vi "FPGA_Master.vi"() -> ()   [LabVIEW 2019]
panel:
  out "Error ?":bool=TRUE
  out "Start sequence?":bool=TRUE
  out "NE cluster":T1
  out "Input Signal / mV":fxp<+/-,19,14> format="%.3g"
  out "Filtered Input":i16(graph)
  out "Filtered Input 2":fxp<+/-,16,16>
  in  "override noise eater?":bool
  in  "Setpoint (H)":fxp<+/-,16,16>
  out "Control Signal / mV":fxp<+/-,19,14> format="%.3g"
  out "Control Signal":i16(graph)
  in  "Setpoint (L)":fxp<+/-,16,16> format="%.3f"
  in  "High power":bool
  in  "Controller output range":T2={"Output high"=10.0, "Output low"=-10.0}
  in  "PID gains":T3={"Proportional gain Kc"=0.0, "Integral time Ti [min]"=2.0, "Derivative time Td [min]"=0.0}
  in  "Reinitialise controller":bool
  out "DIO cluster":T4
  out "AO cluster":T5
  in  "AO7":i16
  in  "AO6":i16
  in  "AO5":i16
  in  "AO4 on":i16
  in  "AO4 off":i16
  in  "AO1 off":i16
  in  "AO1 on":i16
  in  "AO2 off":i16
  in  "AO2 on":i16
  in  "AO3 off":i16
  in  "AO3 on":i16
  in  "AO4":bool
  in  "AO1":bool
  in  "AO3":bool
  in  "AO2":bool
  in  "D31":bool
  in  "D30":bool
  in  "D29":bool
  in  "D28":bool
  in  "D27":bool
  in  "D26":bool
  in  "D25":bool
  in  "D24":bool
  in  "D23":bool
  in  "D22":bool
  in  "D21":bool
  in  "D20":bool
  in  "D19":bool
  in  "D18":bool
  in  "D17":bool
  in  "D16":bool
  in  "D15":bool
  in  "D14":bool
  in  "D13":bool
  in  "D12":bool
  in  "DIO11":bool
  in  "DIO5":bool
  in  "DIO4":bool
  in  "dds/ag":bool
  in  "DIO8":bool
  in  "DIO9":bool
  in  "DIO7":bool
  in  "DIO6":bool
  in  "EOM":bool
  in  "Microwave":bool
  in  "DIO10":bool
  in  "AOM":bool
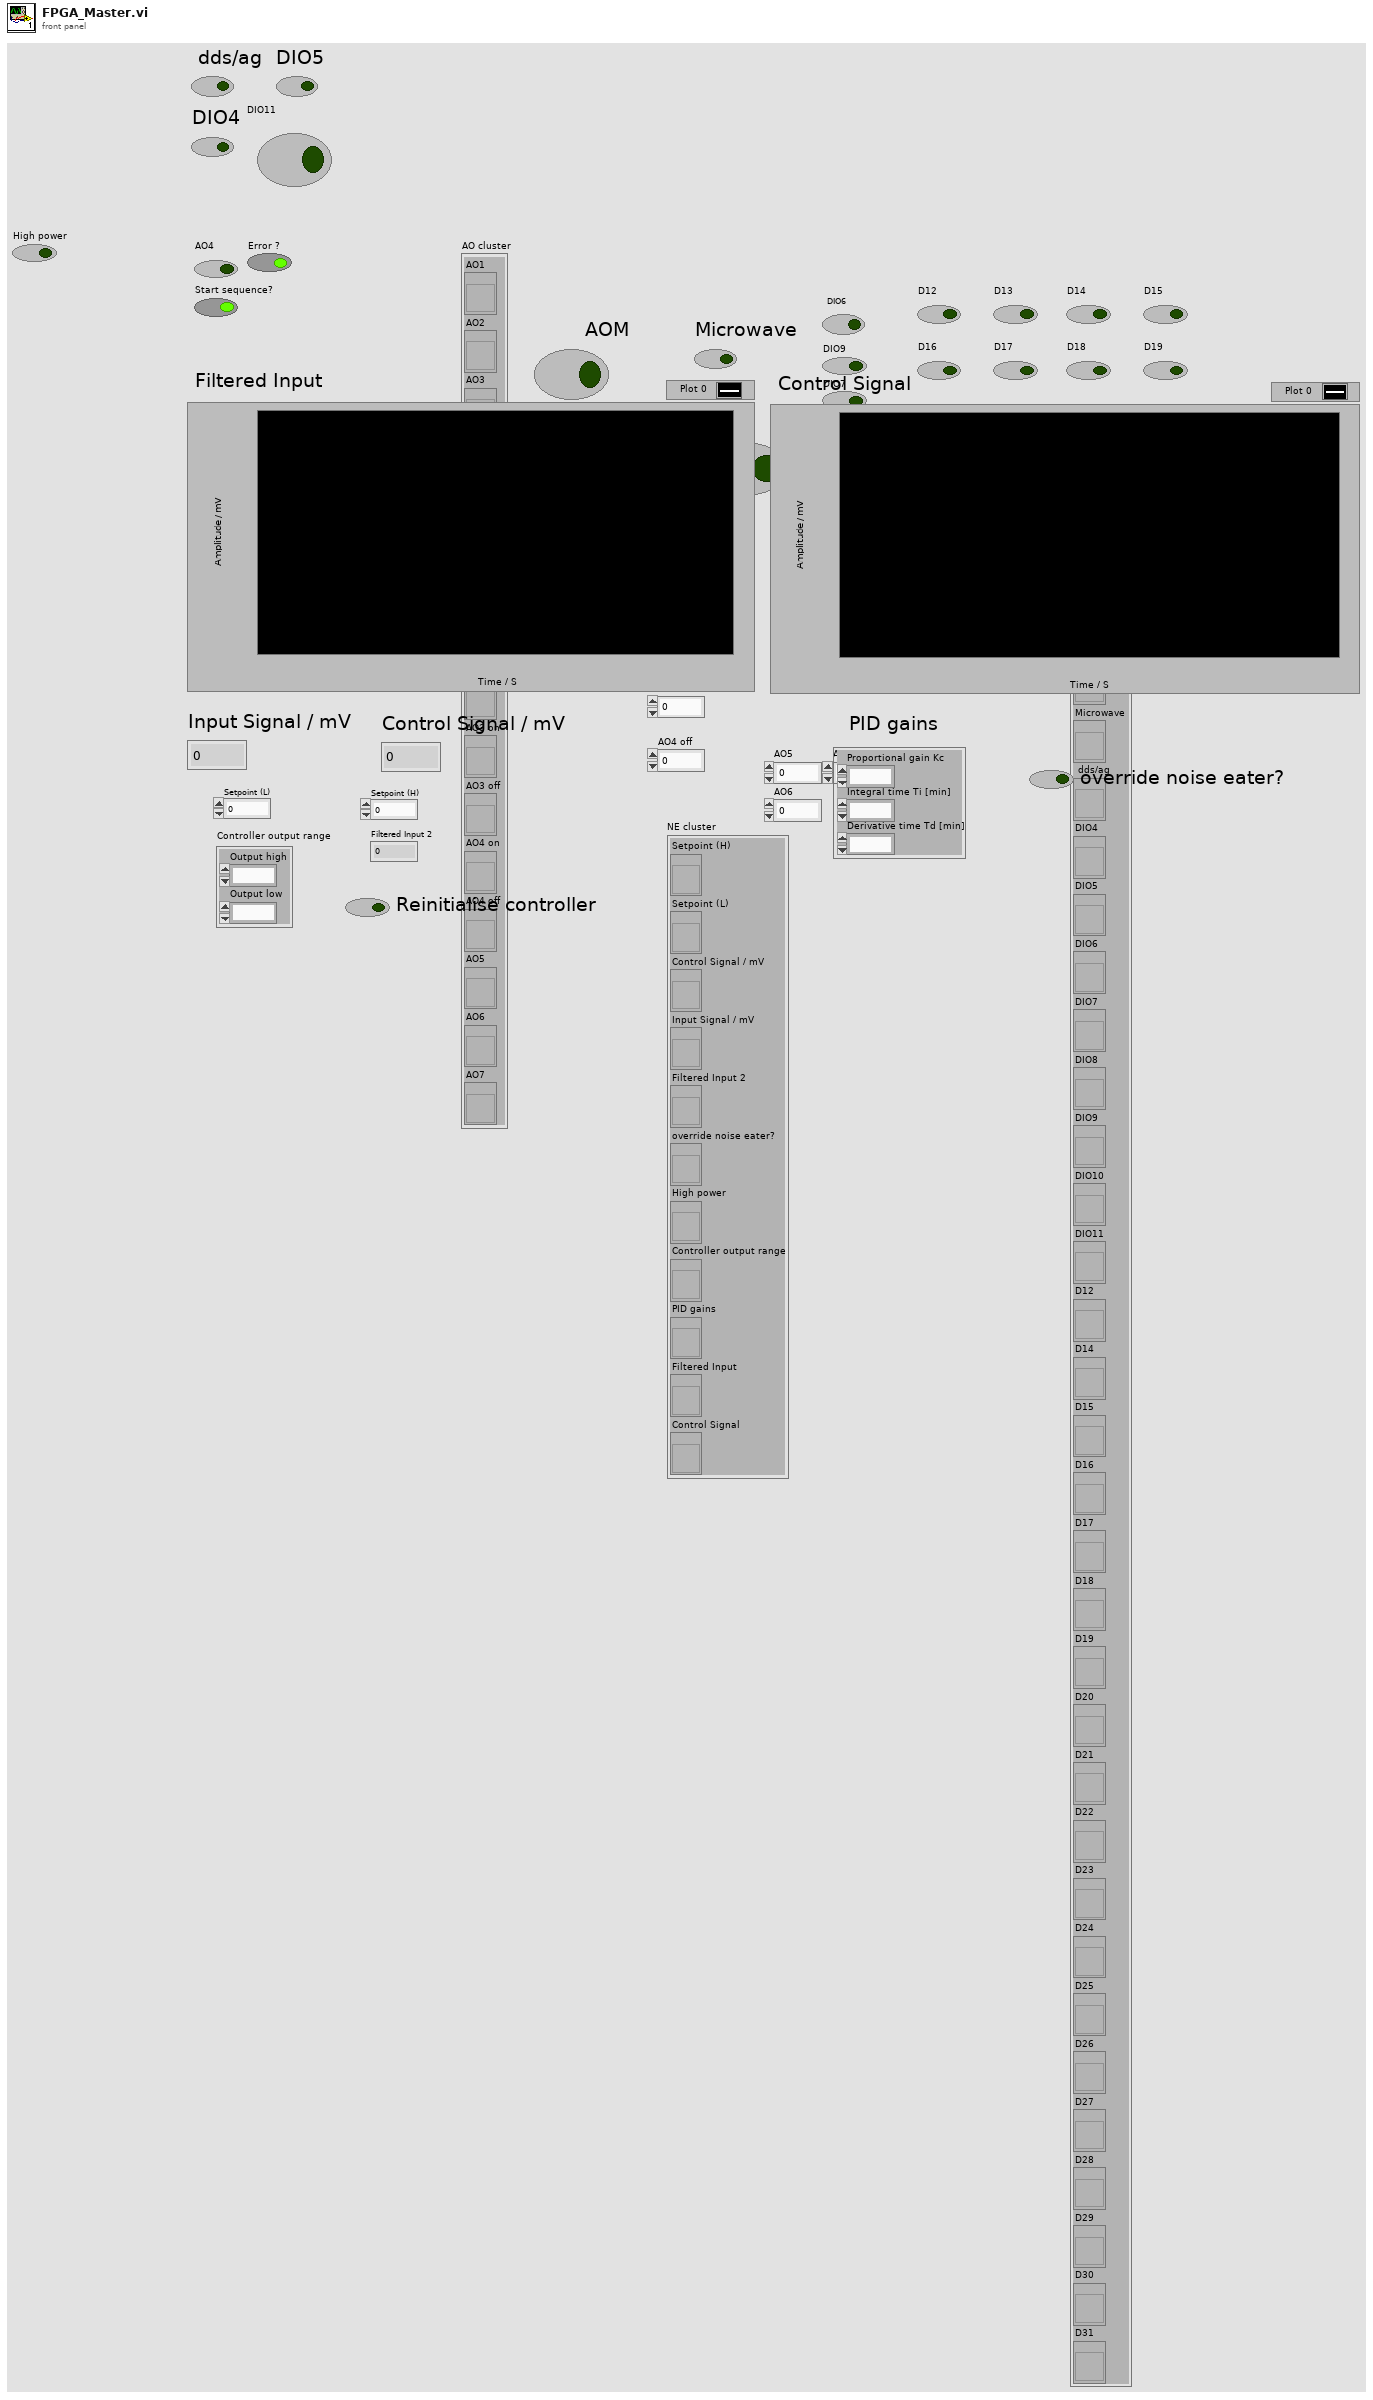
[diagram p1: front panel]
types:
  T1 = cluster{"Setpoint (H)":refnum<vi>, "Setpoint (L)":refnum<vi>, "Control Signal / mV":refnum<vi>, "Input Signal / mV":refnum<vi>, "Filtered Input 2":refnum<vi>, "override noise eater?":refnum<vi>, "High power":refnum<vi>, "Controller output range":refnum<vi>, "PID gains":refnum<vi>, "Filtered Input":refnum<vi>, "Control Signal":refnum<vi>}
  T2 = cluster{"Output high":fxp<+/-,16,16>, "Output low":fxp<+/-,16,16>}
  T3 = cluster{"Proportional gain Kc":fxp<+/-,16,8>, "Integral time Ti [min]":fxp<+/-,16,8>, "Derivative time Td [min]":fxp<+/-,16,8>}
  T4 = cluster{"AOM":refnum<vi>, "EOM":refnum<vi>, "Microwave":refnum<vi>, " dds/ag":refnum<vi>, "DIO4":refnum<vi>, "DIO5":refnum<vi>, "DIO6":refnum<vi>, "DIO7":refnum<vi>, "DIO8":refnum<vi>, "DIO9":refnum<vi>, "DIO10":refnum<vi>, "DIO11":refnum<vi>, "D12":refnum<vi>, "D14":refnum<vi>, "D15":refnum<vi>, "D16":refnum<vi>, "D17":refnum<vi>, "D18":refnum<vi>, "D19":refnum<vi>, "D20":refnum<vi>, "D21":refnum<vi>, "D22":refnum<vi>, "D23":refnum<vi>, "D24":refnum<vi>, "D25":refnum<vi>, "D26":refnum<vi>, "D27":refnum<vi>, "D28":refnum<vi>, "D29":refnum<vi>, "D30":refnum<vi>, "D31":refnum<vi>}
  T5 = cluster{"AO1":refnum<vi>, "AO2":refnum<vi>, "AO3":refnum<vi>, "AO4":refnum<vi>, "AO1 on":refnum<vi>, "AO1 off":refnum<vi>, "AO2 on":refnum<vi>, "AO2 off":refnum<vi>, "AO3 on":refnum<vi>, "AO3 off":refnum<vi>, "AO4 on":refnum<vi>, "AO4 off":refnum<vi>, "AO5":refnum<vi>, "AO6":refnum<vi>, "AO7":refnum<vi>}
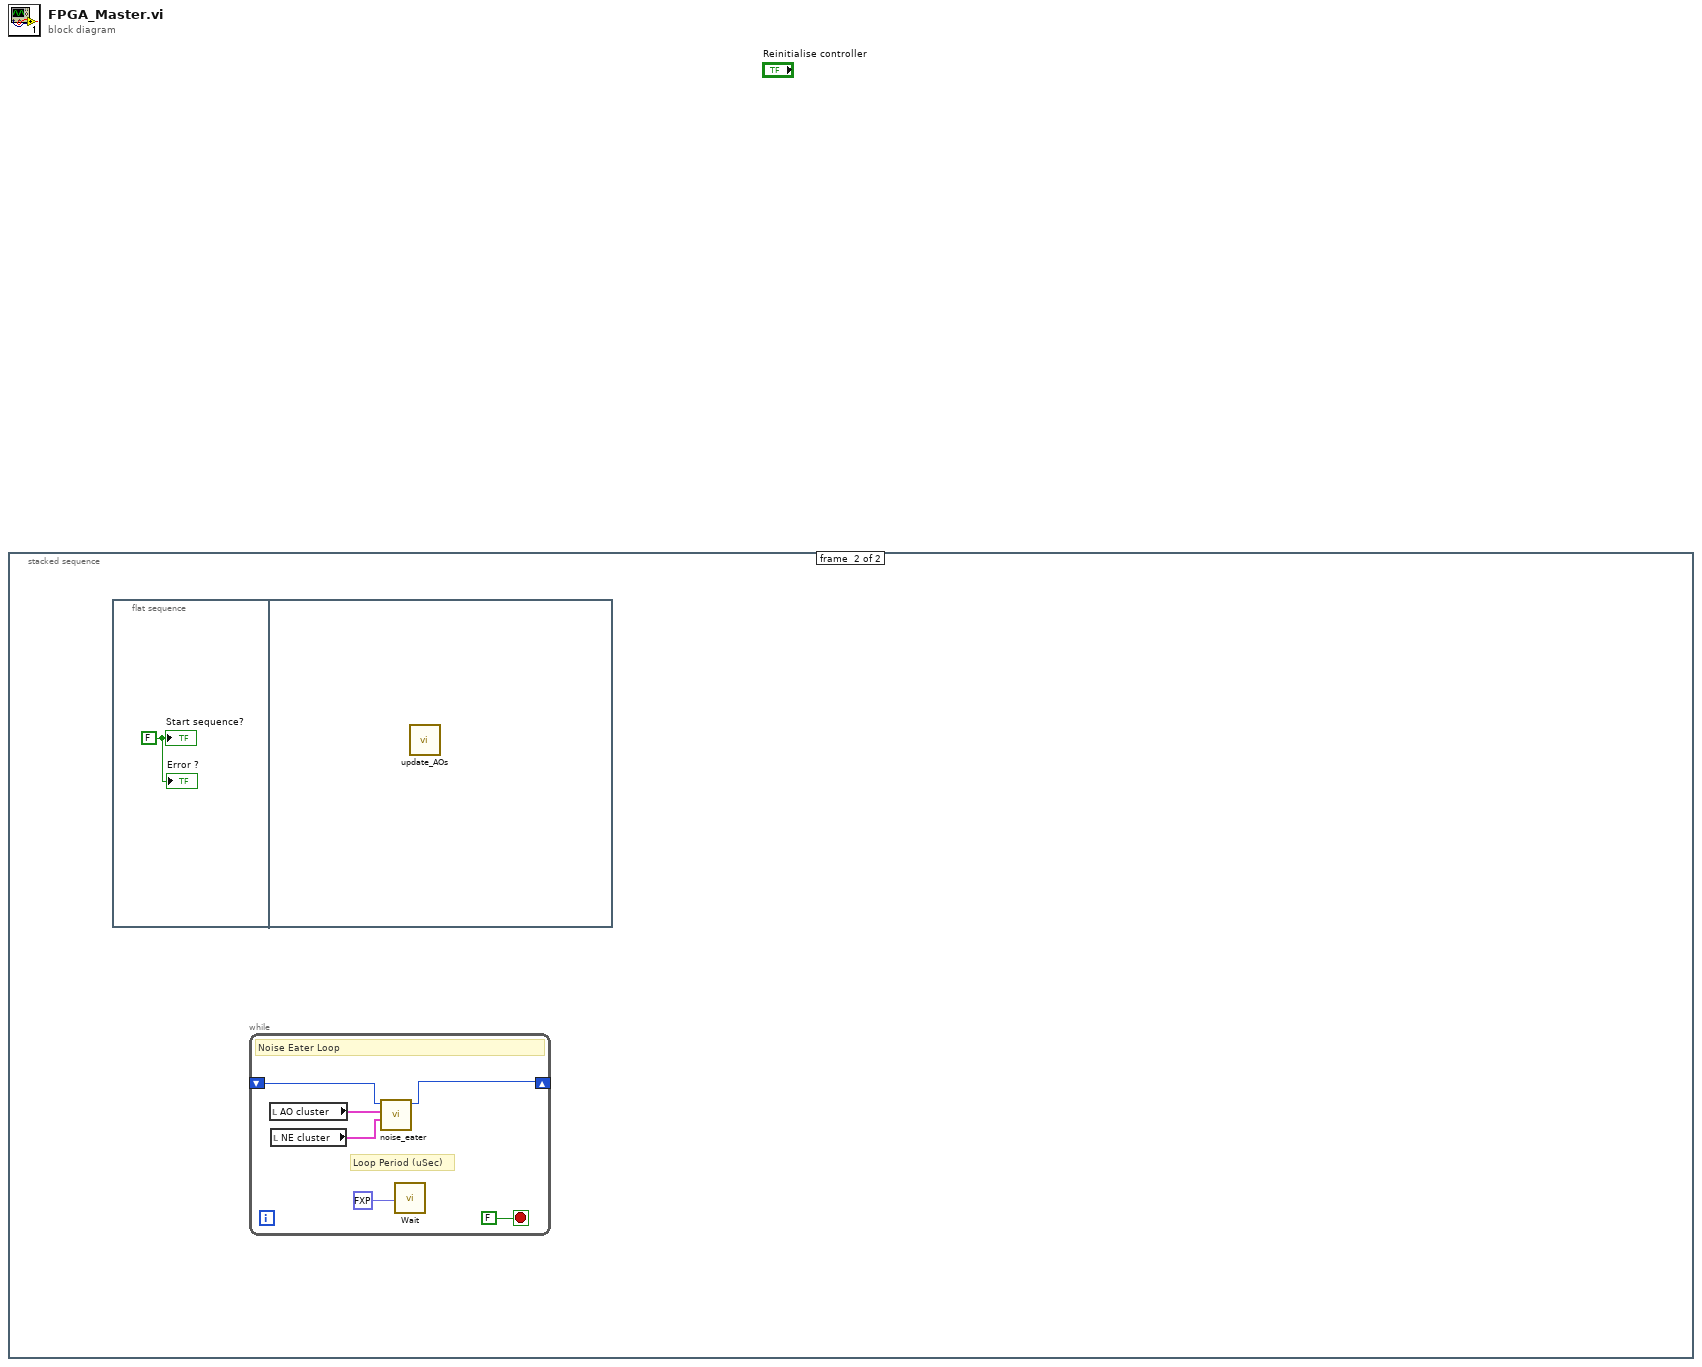
[diagram p0: block diagram]
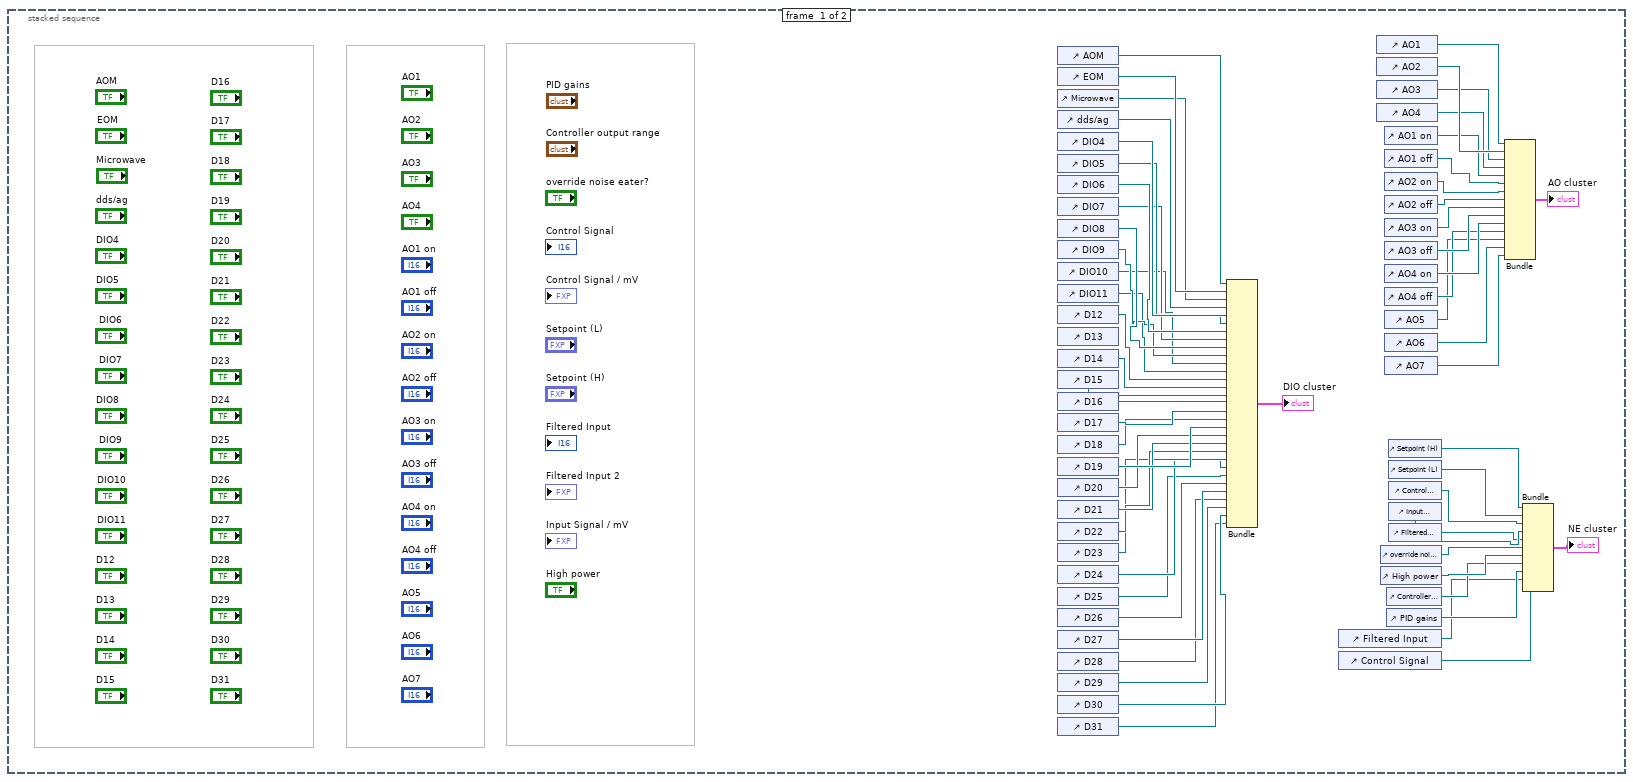
[diagram p2: hidden frame]
diagram:
  n1 = stacked-sequence {
    frame #0 {
      n2 = control-ref of="AOM"() -> (w44:refnum<vi>)
      n3 = control-ref of="EOM"() -> (w43:refnum<vi>)
      n4 = control-ref of="Microwave"() -> (w42:refnum<vi>)
      n5 = control-ref of="dds/ag"() -> (w41:refnum<vi>)
      n6 = control-ref of="DIO4"() -> (w40:refnum<vi>)
      n7 = control-ref of="DIO5"() -> (w39:refnum<vi>)
      n8 = control-ref of="DIO6"() -> (w38:refnum<vi>)
      n9 = control-ref of="DIO7"() -> (w37:refnum<vi>)
      n10 = control-ref of="DIO8"() -> (w36:refnum<vi>)
      n11 = control-ref of="DIO9"() -> (w35:refnum<vi>)
      n12 = control-ref of="DIO10"() -> (w34:refnum<vi>)
      n13 = control-ref of="DIO11"() -> (w33:refnum<vi>)
      n14 = control-ref of="D12"() -> (w32:refnum<vi>)
      n15 = control-ref of="D13"() -> ()  [unwired: 1 out]
      n16 = control-ref of="D14"() -> (w31:refnum<vi>)
      n17 = control-ref of="D15"() -> (w30:refnum<vi>)
      n18 = control-ref of="D16"() -> (w29:refnum<vi>)
      n19 = control-ref of="D17"() -> (w28:refnum<vi>)
      n20 = control-ref of="D18"() -> (w27:refnum<vi>)
      n21 = control-ref of="D19"() -> (w26:refnum<vi>)
      n22 = control-ref of="D20"() -> (w25:refnum<vi>)
      n23 = control-ref of="D21"() -> (w24:refnum<vi>)
      n24 = control-ref of="D22"() -> (w23:refnum<vi>)
      n25 = control-ref of="D23"() -> (w22:refnum<vi>)
      n26 = control-ref of="D24"() -> (w21:refnum<vi>)
      n27 = control-ref of="D25"() -> (w20:refnum<vi>)
      n28 = control-ref of="D26"() -> (w19:refnum<vi>)
      n29 = control-ref of="D27"() -> (w18:refnum<vi>)
      n30 = control-ref of="D28"() -> (w17:refnum<vi>)
      n31 = control-ref of="D29"() -> (w16:refnum<vi>)
      n32 = control-ref of="D30"() -> (w15:refnum<vi>)
      n33 = control-ref of="D31"() -> (w14:refnum<vi>)
      n34 = Bundle("AOM"=w44, "EOM"=w43, "Microwave"=w42, "dds/ag"=w41, "DIO4"=w40, "DIO5"=w39, "DIO6"=w38, "DIO7"=w37, "DIO8"=w36, "DIO9"=w35, "DIO10"=w34, "DIO11"=w33, "D12"=w32, "D14"=w31, "D15"=w30, "D16"=w29, "D17"=w28, "D18"=w27, "D19"=w26, "D20"=w25, "D21"=w24, "D22"=w23, "D23"=w22, "D24"=w21, "D25"=w20, "D26"=w19, "D27"=w18, "D28"=w17, "D29"=w16, "D30"=w15, "D31"=w14) -> (→"DIO cluster":T4)  [unwired: 1 in]
      n35 = control-ref of="Filtered Input"() -> (w3:refnum<vi>)
      n36 = control-ref of="Control Signal"() -> (w2:refnum<vi>)
      n37 = control-ref of="AO1"() -> (w60:refnum<vi>)
      n38 = control-ref of="AO2"() -> (w59:refnum<vi>)
      n39 = control-ref of="AO3"() -> (w58:refnum<vi>)
      n40 = control-ref of="AO4"() -> (w57:refnum<vi>)
      n41 = control-ref of="override noise eater?"() -> (w7:refnum<vi>)
      n42 = control-ref of="High power"() -> (w6:refnum<vi>)
      n43 = control-ref of="AO1 on"() -> (w56:refnum<vi>)
      n44 = control-ref of="AO1 off"() -> (w55:refnum<vi>)
      n45 = control-ref of="AO2 on"() -> (w54:refnum<vi>)
      n46 = control-ref of="AO2 off"() -> (w53:refnum<vi>)
      n47 = control-ref of="AO3 on"() -> (w52:refnum<vi>)
      n48 = control-ref of="AO3 off"() -> (w51:refnum<vi>)
      n49 = control-ref of="AO4 on"() -> (w50:refnum<vi>)
      n50 = control-ref of="AO4 off"() -> (w49:refnum<vi>)
      n51 = control-ref of="AO5"() -> (w48:refnum<vi>)
      n52 = control-ref of="AO6"() -> (w47:refnum<vi>)
      n53 = control-ref of="AO7"() -> (w46:refnum<vi>)
      n54 = control-ref of="Controller output range"() -> (w5:refnum<vi>)
      n55 = control-ref of="PID gains"() -> (w4:refnum<vi>)
      n56 = control-ref of="Setpoint (H)"() -> (w12:refnum<vi>)
      n57 = control-ref of="Setpoint (L)"() -> (w11:refnum<vi>)
      n58 = control-ref of="Control Signal / mV"() -> (w10:refnum<vi>)
      n59 = control-ref of="Input Signal / mV"() -> (w9:refnum<vi>)
      n60 = control-ref of="Filtered Input 2"() -> (w8:refnum<vi>)
      n61 = Bundle("AO1"=w60, "AO2"=w59, "AO3"=w58, "AO4"=w57, "AO1 on"=w56, "AO1 off"=w55, "AO2 on"=w54, "AO2 off"=w53, "AO3 on"=w52, "AO3 off"=w51, "AO4 on"=w50, "AO4 off"=w49, "AO5"=w48, "AO6"=w47, "AO7"=w46) -> (→"AO cluster":T5)  [unwired: 1 in]
      n62 = Bundle("Setpoint (H)"=w12, "Setpoint (L)"=w11, "Control Signal / mV"=w10, "Input Signal / mV"=w9, "Filtered Input 2"=w8, "override noise eater?"=w7, "High power"=w6, "Controller output range"=w5, "PID gains"=w4, "Filtered Input"=w3, "Control Signal"=w2) -> (→"NE cluster":T1)  [unwired: 1 in]
    }
    frame #1 {
      n63 = flat-sequence {
        frame #0 {
          w61 = FALSE ("Start sequence?")
          "Start sequence?" <- w61
          "Error ?" <- w61
        }
        frame #1 {
          n64 = call "update_AOs.vi"() -> ()  [unwired: 12 in]
        }
      }
      n65 = while {
        shift-right: [w62] -> _
        shift-left: _ -> [w63]
        stop <- FALSE stop-if-true
        # "Loop Period (uSec)"
        # "Noise Eater Loop"
        n66 = local read "AO cluster"() -> (w67:T5)
        n67 = local read "NE cluster"() -> (w66:T1)
        n68 = call "noise_eater.vi"("In val"=w63, "AO cluster"=w67, "NE cluster"=w66) -> ("Out val"=w62:i16)  [unwired: 7 in]
        n69 = call "Wait"("Count(uSec)"=fxp<+,1,4> 8.0) -> ()  [unwired: 1 out]
      }
    }
  }
